vi "AODScanner_5_May_2014.vi"() -> ()   [LabVIEW 2012]
uses:
  AODAcq/AODAcq.lvclass
  <vilib>/rvi/interface/nirviReadWriteControl/nirviReadWriteControl.xnode
  FPGA_Control/AODRef.ctl
  <vilib>/rvi/interface/nirviMethod/nirviMethod.xnode
  <vilib>/rvi/errors/niLvFpgaMergeErrorWithErrorCode.vi
  Motion Stabilization/GlobalVars.vi
  <vilib>/DAQmx/write.llb/DAQmx Write (Analog DBL 1Chan 1Samp).vi
  <vilib>/DAQmx/read.llb/DAQmx Read (Analog Wfm 1Chan NSamp).vi
panel:
  out "Motion FIFO":refnum<queue>
  out "Motion ROIs":T1(array[cluster])
  out "Motion Plane Centers":i32[][](array[numeric])
  out "Number of Motion Planes":i32
  in  "Motion rate (Hz) 2":dbl=10.0
  out "error out 3":errorcluster
  out "Out Points":i32[][](array[numeric])
  out "Y-Z Motion Points":i32[][](array[numeric])
  out "X-Y Motion Points":i32[][](array[numeric])
  out "Points_um":dbl[][](array[numeric])
  out "Lens Magnification":i32=20
  in  "Matlab Server Shared Folder":string="c:\\temp"
  in  "Matlab Server IP Address":string="10.21.16.18"
  in  "External Magnification":dbl=1.3
  out "error out 2":errorcluster
  out "Objective Position":cluster{"X":dbl, "Y":dbl, "Z":dbl}
  out "Numeric":i32=299
  out "error out":errorcluster
  out "ROIs":T1(array[cluster])
  out "Histogram":dynamicdata(graph)
  out "Raw samples remaining":u32
  out "Temporal samples remaining":u32
  out "Motion samples remaining":u32
  out "Image samples remaining":u32
  out "Recording File":path
  out "Waveform Chart":waveform(dbl)(graph)
  out "Ephys":bool
  in  "TraceElements":u32=10000
  out "ScanProgress":dbl(slide) scale=0.0..1.0
  in  "Abort":bool
  out "Progress":dbl(slide) scale=0.0..1.0
  in  "SweepSettings":bool
  in  "stop":bool
  in  "Power":dbl(slide)=2.5 min=0.0 max=5.0 step=0.1 scale=0.0..2.5
  out "Scan":bool
  out "Volume":bool
  in  "Tab Control":enum32{"Setup", "Volume", "Traces", "Motion"}(tab)
  in  "Store Raw":bool
  in  "Disp Volume":bool=TRUE
  in  "Save Volume":bool
  in  "Ephys":bool
  in  "Motion rate (Hz)":dbl=10.0
  in  "Scan Settings (um)":T2={"XStart"=-100, "XEnd"=100, "XNum"=250, "YStart"=-100, "YEnd"=100, "YNum"=250, "ZStart"=-30, "ZEnd"=70, "ZNum"=60}
  in  "Objective":enum16{"20x Olympus"}(ring)
  in  "Scan Time (s)":dbl=300.0
  in  "Volume Reps":i32=1 min=1 max=10000
  in  "Volume":bool
  in  "Scan":bool
  in  "Motion Channel To Analyze":i32=2 min=1 max=2
  in  "Motion Analysis":bool
  in  "Per Cell Motion Analysis":bool
  in  "Sampling Structure":u16(ring) items=["Cube Vertices"]
  in  "Motion Box Params":T3={"XY Offset"=3, "Z Offset"=6, "Line Length"=12.0, "Box Size"=12.0}
  in  "ClearMotionCenters":bool
  in  "Point Centering":bool=TRUE
  in  "Recenter":bool caption="OK Button"
  out "Motion Points (Ch1)":u32
  out "Number selected":u32
  in  "Contrast":dbl(slide)=99.63636363636364 scale=98.0..100.0
  out "ImCh2":T4(plugin-control)
  out "ImCh1":T4(plugin-control)
  in  "Section":dbl min=0.0 max=59.0 step=1.0
  in  "Segment":bool
  out "Motion Increment":u32
  in  "Offset":dbl(slide)=0.010101010101010102 scale=0.0..1.0
  in  "ClearPoints":bool
  out "Total Motion Points":i32
  out "Motion Ch1":T4(plugin-control)
  out "Ephys":waveform(dbl)[](graph)
  out "Traces":waveform(dbl)[](graph)
  in  "Down Rate":i32=500
  in  "Spacing":dbl=100.0
  in  "Decimate":bool
  in  "Baseline Offset":dbl
  out "Motion Ch2":T4(plugin-control)
  out "Finished":bool
  out "Stopped":bool
  out "AODAcq out":refnum<class "AODAcq.lvclass">
  in  "Debug":bool
  in  "GridPoints":u16=10
  out "Scan Settings":T2
  out "VolData":i32[][](array[numeric])
  in  "VolumeElements":u32=10000
  in  "Points":i32[][](array[numeric])
  # "Off"
  # "On"
  # "On"
  # "Off"
  # "Off"
  # "On"
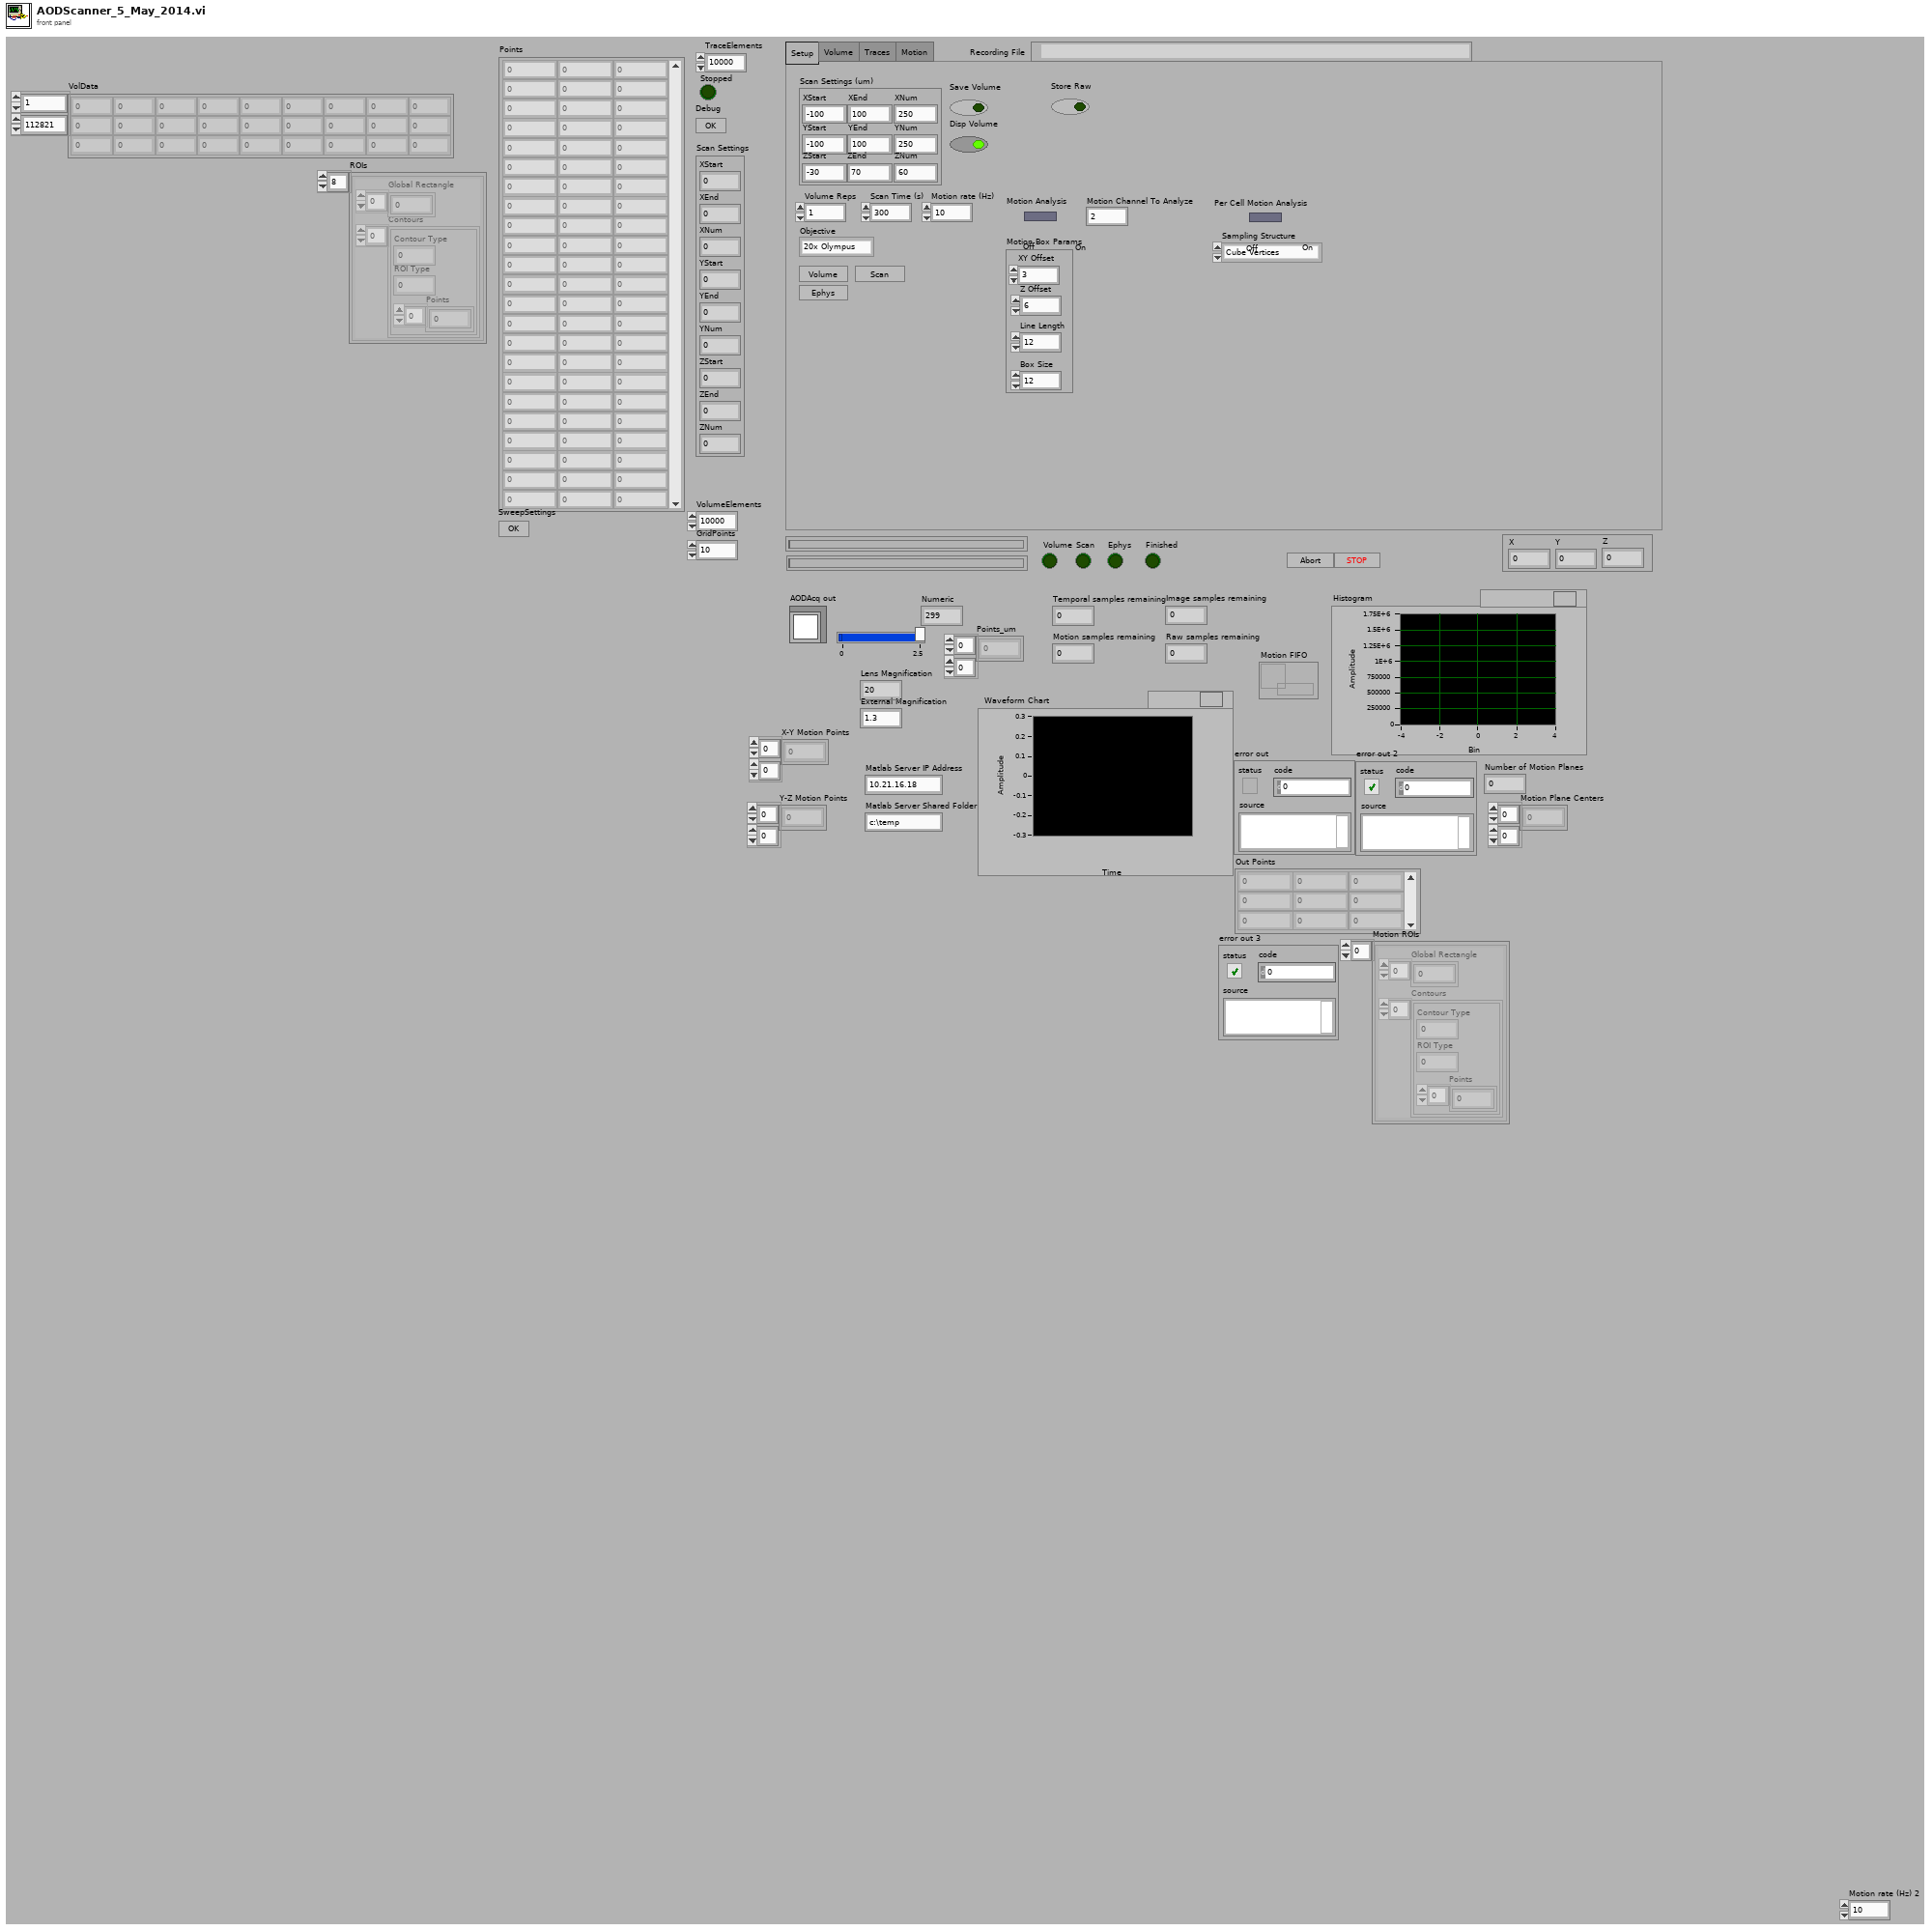
[diagram p1: front panel]
types:
  T1 = cluster{"Global Rectangle":i32[], "Contours":cluster{"Contour Type":u32, "ROI Type":u32, "Points":i32[]}[]}[]
  T2 = cluster{"XStart":i32, "XEnd":i32, "XNum":i32, "YStart":i32, "YEnd":i32, "YNum":i32, "ZStart":i32, "ZEnd":i32, "ZNum":i32}
  T3 = cluster{"XY Offset":i32, "Z Offset":i32, "Line Length":dbl, "Box Size":dbl}
  T4 = typedef "IMAQ Image.ctl" = refnum<image>
  T5 = typedef "Image Type" = u32
  T6 = cluster{"Global Rectangle":i32[], "Contours":cluster{"Contour Type":u32, "ROI Type":u32, "Points":i32[]}[]}
  T7 = cluster{"queue out":refnum<queue>, "queue out":refnum<queue>, "queue out":refnum<queue>}
  T8 = typedef "AODRef.ctl" = refnum<k20>
  T9 = cluster{"Scan Settings":cluster{"XStart":i32, "XEnd":i32, "XNum":i32, "YStart":i32, "YEnd":i32, "YNum":i32, "ZStart":i32, "ZEnd":i32, "ZNum":i32}, "Scan Settings (um)":cluster{"XStart":i32, "XEnd":i32, "XNum":i32, "YStart":i32, "YEnd":i32, "YNum":i32, "ZStart":i32, "ZEnd":i32, "ZNum":i32}}
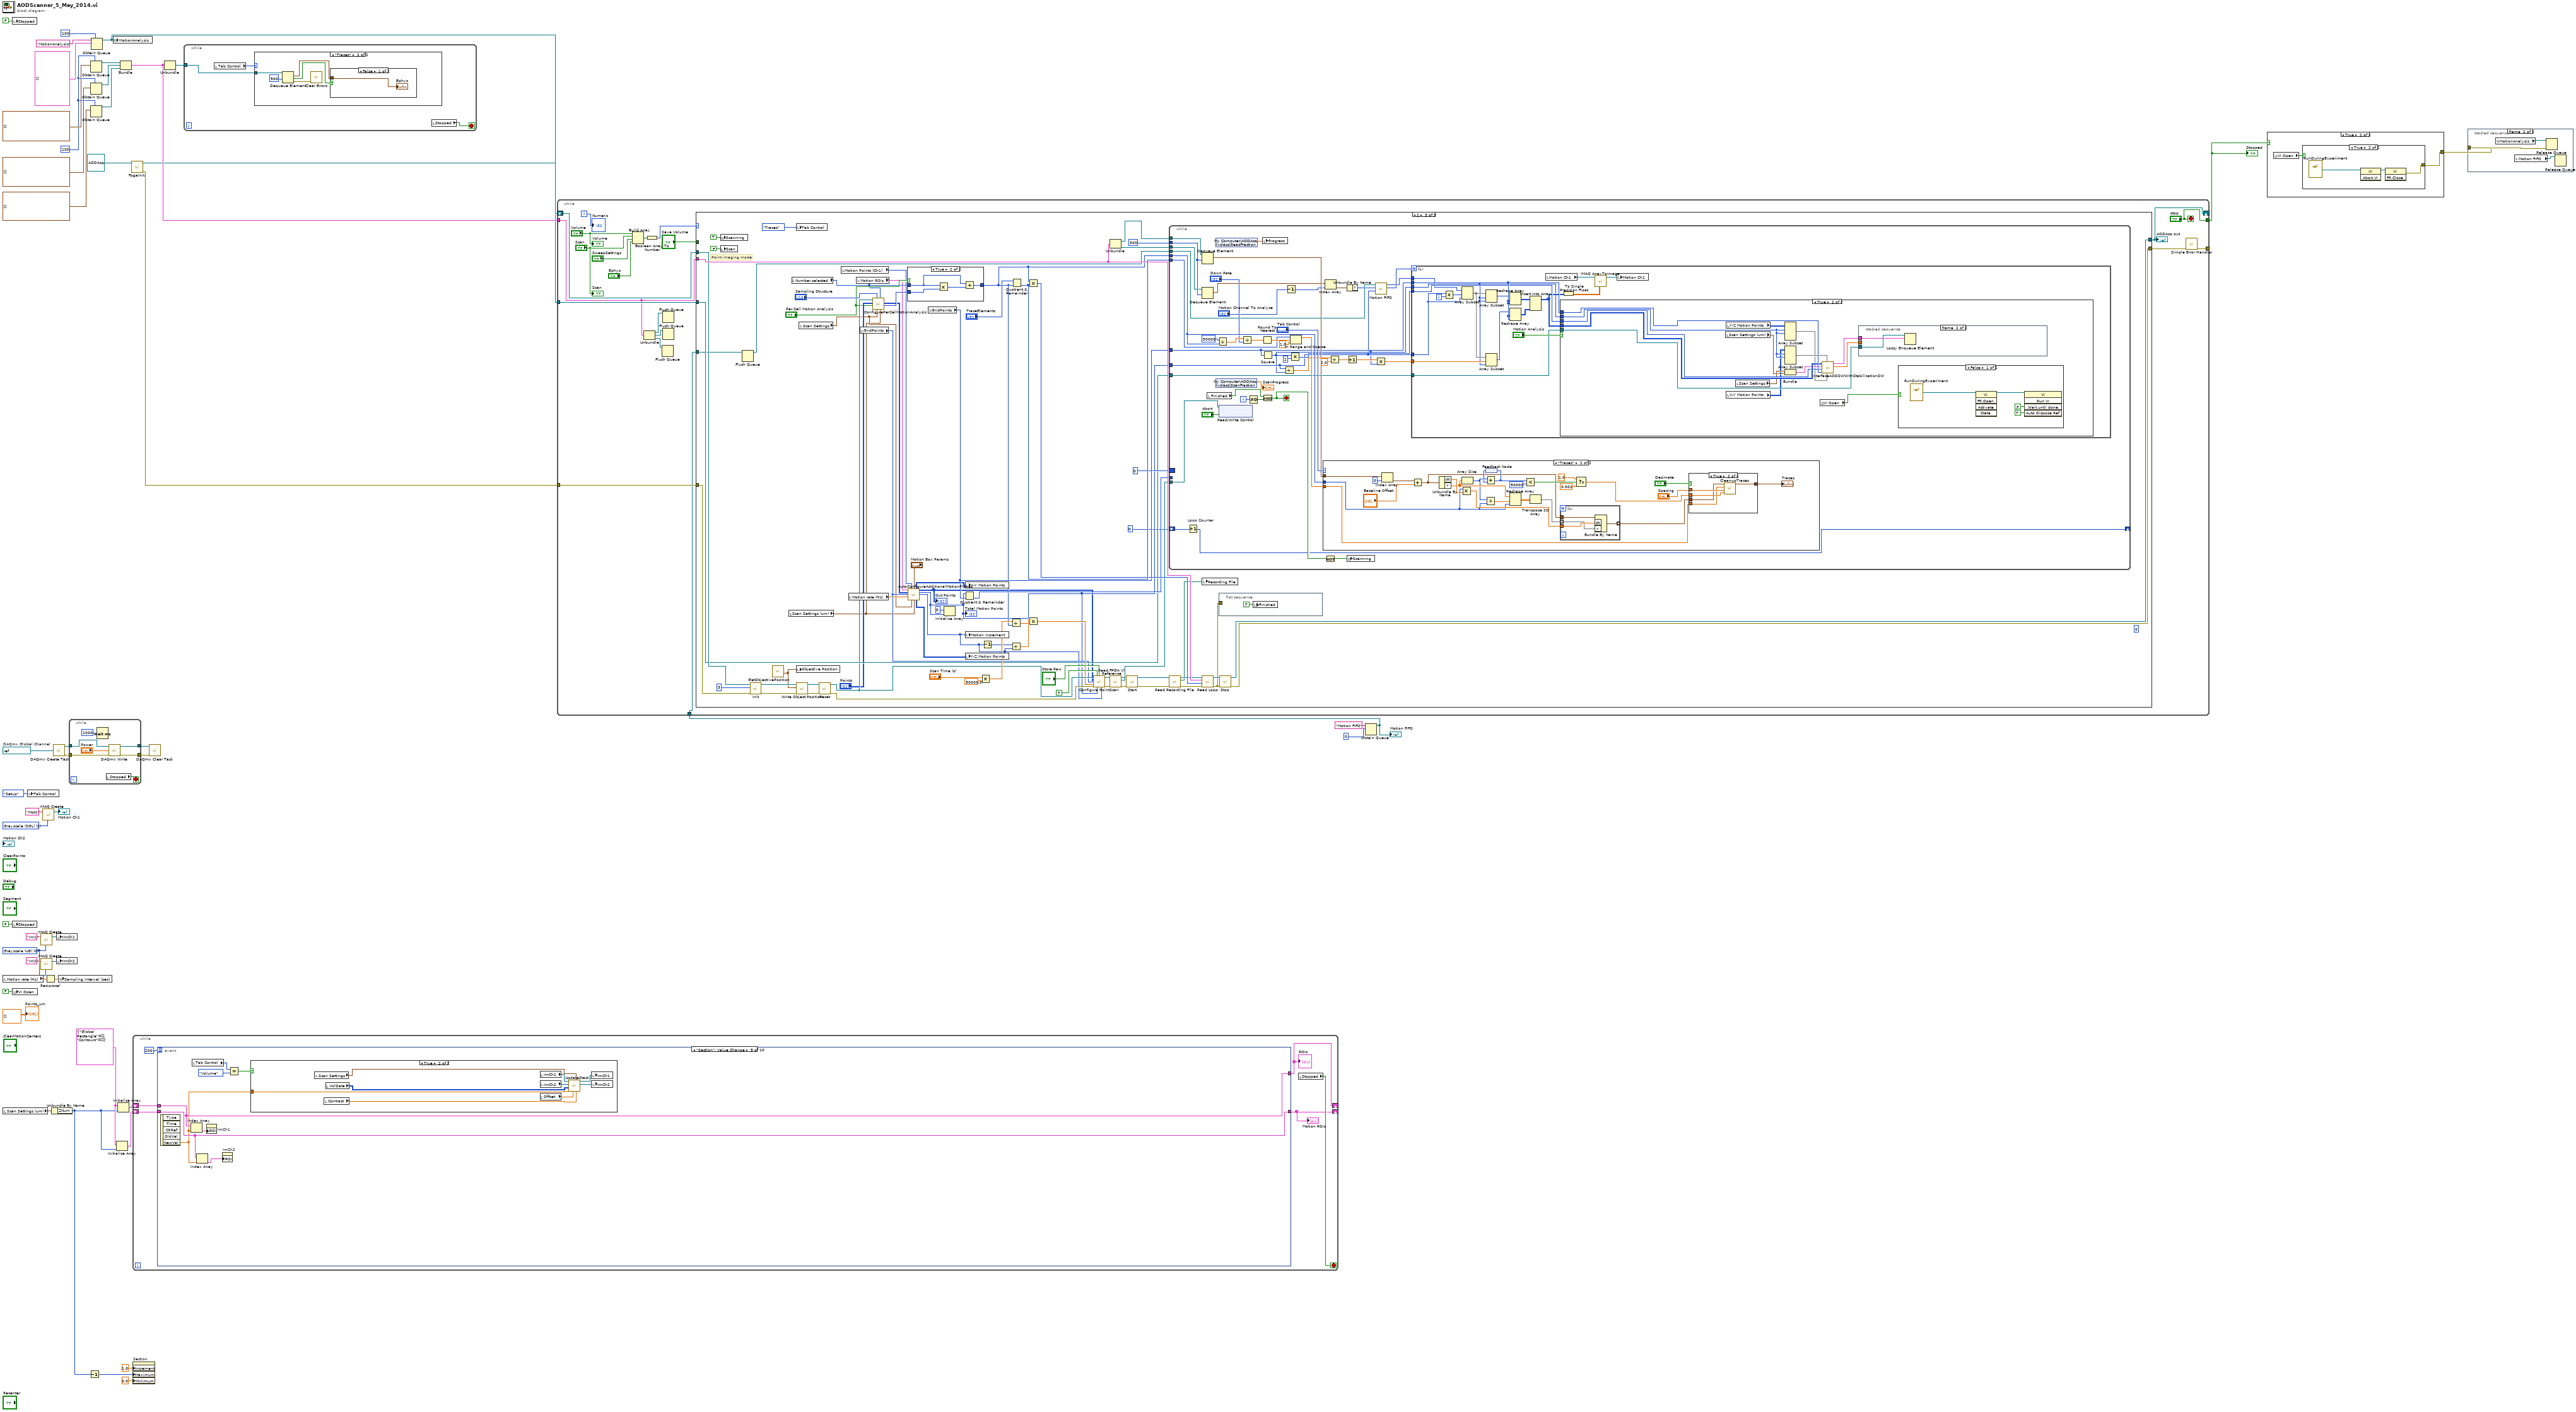
[diagram p0: block diagram]
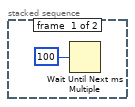
[diagram p2: hidden frame]
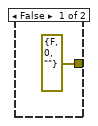
[diagram p3: hidden frame]
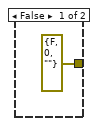
[diagram p4: hidden frame]
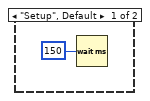
[diagram p5: hidden frame]
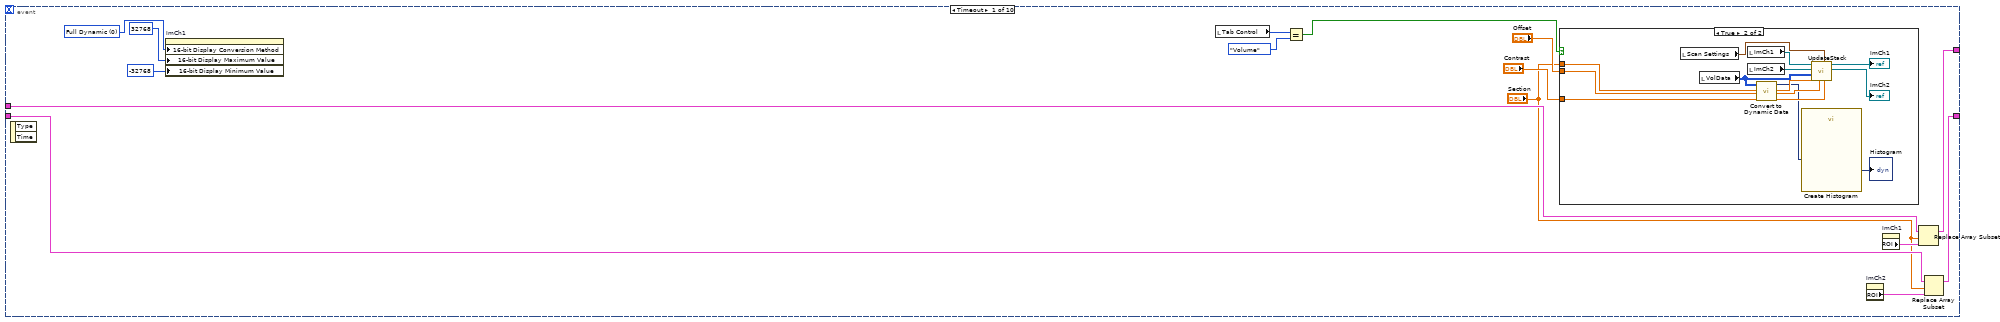
[diagram p7: hidden frame]
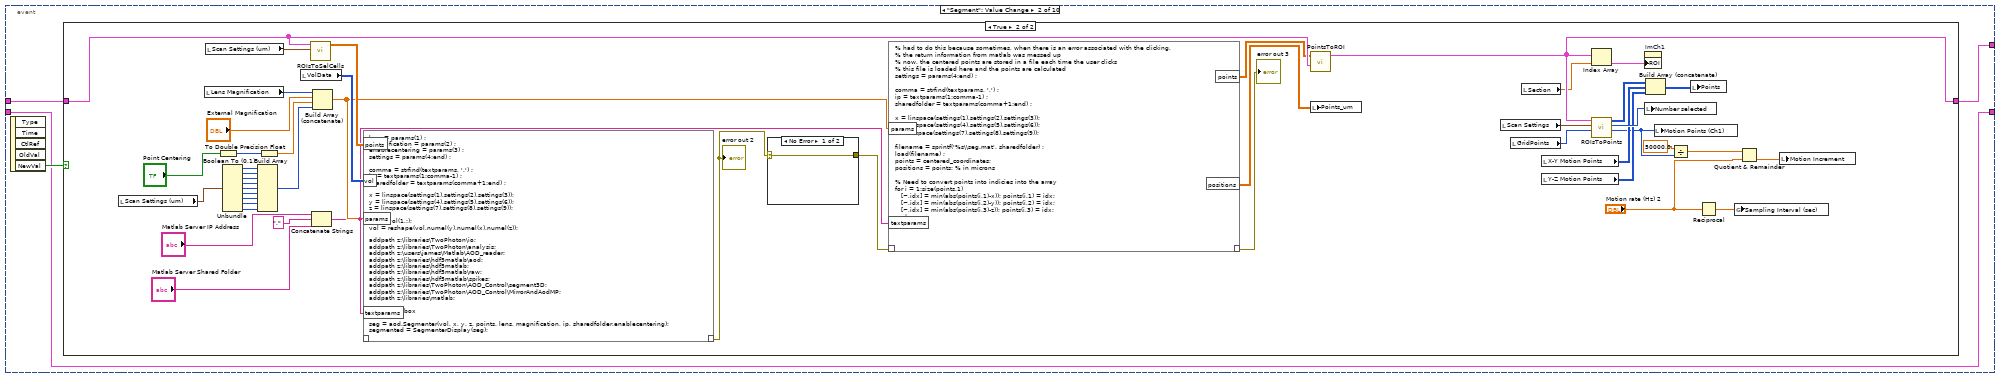
[diagram p9: hidden frame]
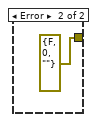
[diagram p11: hidden frame]
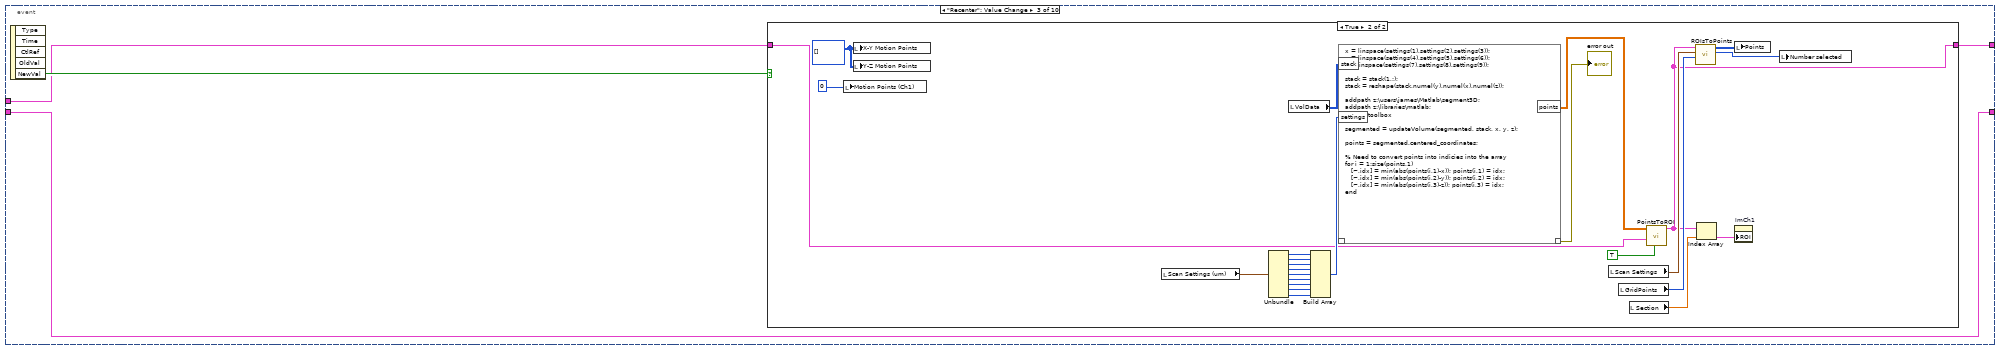
[diagram p12: hidden frame]
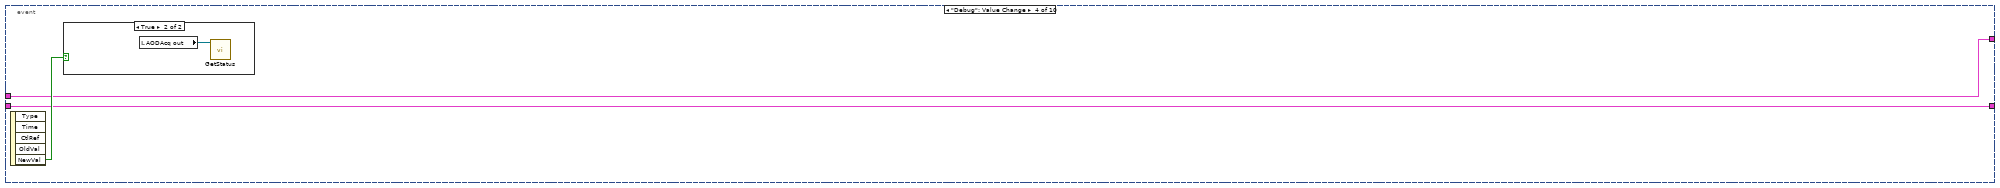
[diagram p14: hidden frame]
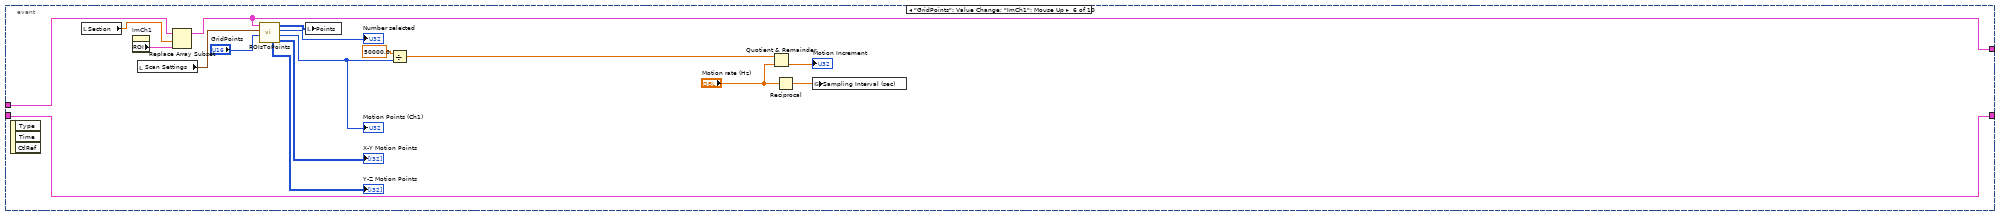
[diagram p17: hidden frame]
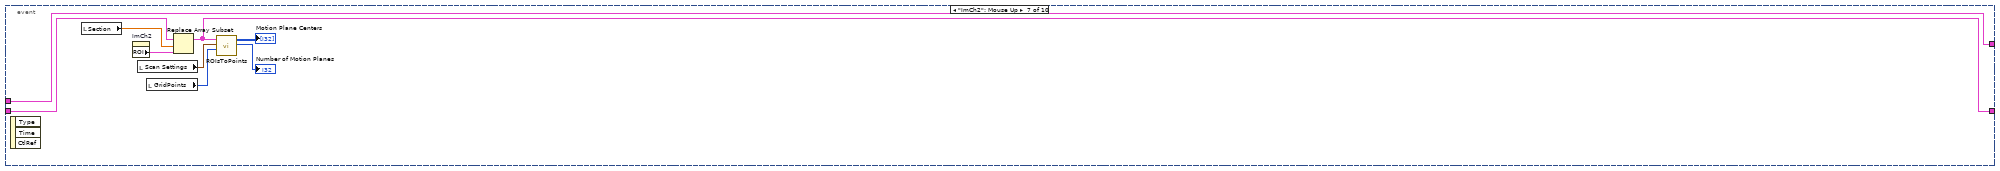
[diagram p18: hidden frame]
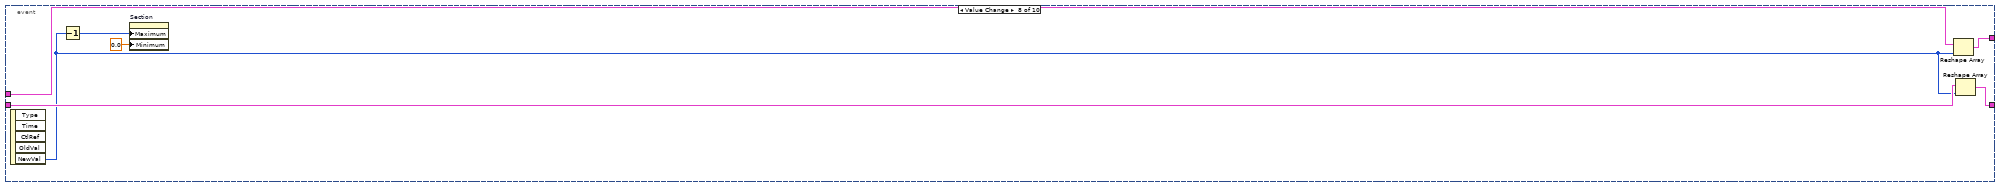
[diagram p19: hidden frame]
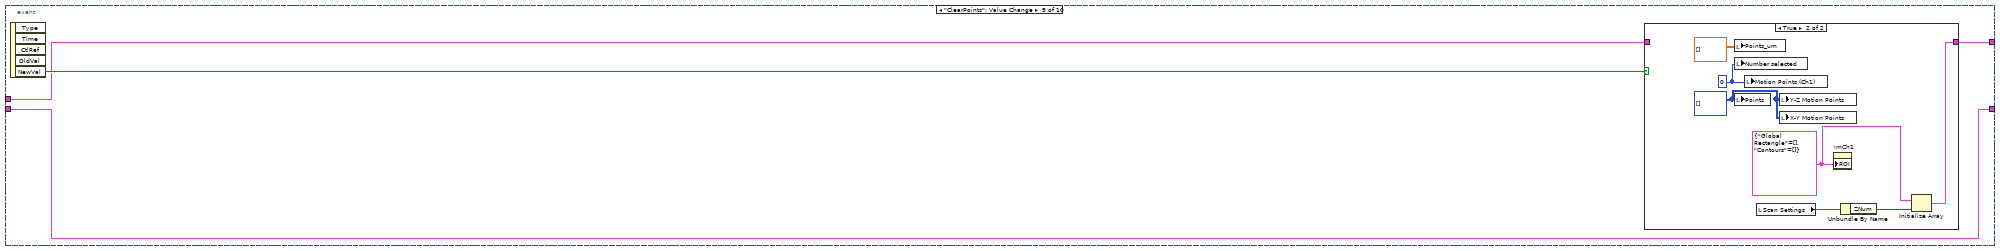
[diagram p20: hidden frame]
diagram:
  w18 = 100 ("max queue size (-1, unlimited)")
  w23 = T5 2 items=["Grayscale (U8)", "Grayscale (I16)", "Grayscale (SGL)", "Complex (CSG)", "RGB (U32)", "HSL (U32)", "RGB (U64)", "Grayscale (U16)"] ("Image Type")
  w34 = T5 0 items=["Grayscale (U8)", "Grayscale (I16)", "Grayscale (SGL)", "Complex (CSG)", "RGB (U32)", "HSL (U32)", "RGB (U64)", "Grayscale (U16)"] ("Image Type")
  w6 = T6 {"Global Rectangle"=[], "Contours"=[]} ("ROI")
  w44 = refnum<k21> "AOD Gain"  # DAQmx Global Channel
  n1 = local read "Motion rate (Hz)"() -> (w9:dbl)
  n2 = local read "Scan Settings (um)"() -> (w38:T2)
  n3 = local write "Stopped"(FALSE ("Stopped")) -> ()
  n4 = local write "Stopped"(FALSE ("Stopped")) -> ()
  n5 = global write "GlobalVars.vi" "VI Open"(FALSE ("VI Open")) -> ()
  n6 = local write "Tab Control"(enum32{"Setup", "Volume", "Traces", "Motion"}."Setup" ("Tab Control")) -> ()
  n7 = call "IMAQ Create"("Image Name"="Im1", "Image Type"=w34) -> ("New Image"=w46:T4)  [unwired: 3 in, 1 out]
  n8 = call "IMAQ Create"("Image Name"="Im2", "Image Type"=w34) -> ("New Image"=w45:T4)  [unwired: 3 in, 1 out]
  n9 = call "IMAQ Create"("Image Name"="Mot1", "Image Type"=w23) -> ("New Image"=→"Motion Ch1":T4)  [unwired: 3 in, 1 out]
  n10 = Reciprocal(x=w9) -> (1/x=w8:dbl)
  n11 = Unbundle By Name(w38) -> ("ZNum"=w5:i32)
  n12 = call <vilib>:"DAQmx Create Task.vi"("global virtual channels"=w44) -> ("task out"=w43:refnum<k21>, "error out"=w42:errorcluster)  [unwired: 4 in, 9 out]
  n13 = local write "ImCh1"(w46) -> ()
  n14 = local write "ImCh2"(w45) -> ()
  n15 = global write "GlobalVars.vi" "Sampling Interval (sec)"(w8) -> ()
  n16 = while {
    tunnel: w43 -> [w55]
    tunnel: w42 -> [w54]
    tunnel: [w53] -> w41
    tunnel: [w52] -> w40
    stop <- w51 stop-if-true
    n17 = Wait (ms)(milliseconds to wait=u32 1000) -> ()  [unwired: 1 out]
    n18 = local read "Stopped"() -> (w51:bool)
    n19 = call-poly <vilib>:"DAQmx Write.vi"("task/channels in"=w55, "data"="Power", "error in"=w54) -> ("task out"=w53:refnum<k21>, "error out"=w52:errorcluster)  [unwired: 10 in, 1 out]
  }
  n20 = Decrement(x=w5) -> (x-1=w33:i32)
  n21 = Obtain Queue(max queue size (-1, unlimited)=w18, element data type=waveform(i32)[] []) -> (queue out=w29:refnum<queue>)  [unwired: 3 in, 2 out]
  n22 = Obtain Queue(max queue size (-1, unlimited)=w18, element data type=waveform(dbl)[] []) -> (queue out=w30:refnum<queue>)  [unwired: 3 in, 2 out]
  n23 = Obtain Queue(max queue size (-1, unlimited)=w18, element data type=waveform(i32)[] []) -> (queue out=w28:refnum<queue>)  [unwired: 3 in, 2 out]
  n24 = Obtain Queue(max queue size (-1, unlimited)=100, name (unnamed)="MotionAnalysis", element data type=cluster{dbl[][], dbl, dbl, dbl, dbl, dbl, dbl}[] [] ("Array 2")) -> (queue out=w12:refnum<queue>)  [unwired: 2 in, 2 out]
  n25 = global write "GlobalVars.vi" "MotionAnalysis"(w12) -> ()
  n26 = Initialize Array(w6, w5) -> (w4:T1)
  n27 = Initialize Array(w6, w5) -> (w37:T1)
  n28 = Bundle("queue out"=w29, "queue out"=w30, "queue out"=w28) -> (w27:T7)  [unwired: 1 in]
  n29 = call-dynamic "FpgaInit.vi"("AODAcq in"=refnum<class "AODAcq.lvclass"> refnum ("AODAcq.lvclass")) -> ("error out"=w21:errorcluster, "AODAcq out"=w20:refnum<class "AODAcq.lvclass">)  [unwired: 9 in]
  n30 = while {
    shift-right: [w61] -> _
    shift-left: w37 -> [w62]
    shift-right: [w58] -> _
    shift-left: w4 -> [w57]
    stop <- w59 stop-if-true
    n31 = event shown="[4] \"Section\": Value Change" {
      selector: _ -> [_ _ _ _ _ _ _ _ _ _]
      dyn-events: _ -> [_ _ _ _ _ _ _ _ _ _]
      timeout: 200 -> [_ _ _ _ _ _ _ _ _ _]
      tunnel: w62 -> [w76 w91 w143 w173 w182 w209 w210 w223 w227 w239]
      tunnel: [w77 w90 w144 w173 w182 w206 w210 w222 w228 w239] -> w61
      tunnel: [w63 w89 w142 w172 w177 w193 w211 w219 w226 w240] -> w58
      tunnel: w57 -> [w66 w89 w142 w172 w177 w193 w216 w221 w226 w238]
      event Timeout {
        w71 = u32 0 items=["Full Dynamic", "Downshift", "Given Range", "90% Dynamic", "Given Percent Range"] ("16-bit Display Mapping:Conversion Method")
        n32 = event-data() -> ()  [unwired: 1 in, 2 out]
        n33 = property on="ImCh1" class="ImageControl"("16-bit Display Conversion Method"=w71, "16-bit Display Maximum Value"=32768 ("16-bit Display Mapping:Maximum Value"), "16-bit Display Minimum Value"=-32768 ("16-bit Display Mapping:Maximum Value")) -> ()  [unwired: 2 in, 2 out]
        n34 = local read "Tab Control"() -> (w74:enum32{"Setup", "Volume", "Traces", "Motion"})
        n35 = Equal?(x=w74, y=enum32{"Setup", "Volume", "Traces"}."Volume") -> (x = y?=w72:bool)
        n36 = case shown="True" w72 {
          tunnel: "Section" -> [_ w83]
          tunnel: "Offset" -> [_ w82]
          tunnel: "Contrast" -> [_ w81]
          frame False {
          }
          frame True {
            n37 = local read "Scan Settings"() -> (w84:T2)
            n38 = local read "VolData"() -> (w80:i32[][])
            n39 = local read "ImCh1"() -> (w88:T4)
            n40 = local read "ImCh2"() -> (w87:T4)
            n41 = call "Convert to Dynamic Data"("2D Array"=w80) -> ("Dynamic Data Type"=w79:dynamicdata)  [unwired: 3 in]
            n42 = call "Create Histogram"("Signal"=w79) -> ("Histogram"=→"Histogram":dynamicdata)  [unwired: 9 in, 1 out]
            n43 = call "UpdateStack.vi"("Contrast"=w81, "Scan Settings"=w84, "Offset"=w82, "Section"=w83, "ImData"=w80, "Im2 2"=w87, "Im1 In"=w88) -> ("Im2 Out"=→"ImCh2":T4, "Im1 Out"=→"ImCh1":T4)  [unwired: 3 in]
          }
        }
        n44 = property on="ImCh2" class="ImageControl"() -> ("ROI"=w65:T6)  [unwired: 2 in, 2 out]
        n45 = property on="ImCh1" class="ImageControl"() -> ("ROI"=w75:T6)  [unwired: 2 in, 2 out]
        n46 = Replace Array Subset(array=w76, new element=w75, index="Section") -> (w77:T1)
        n47 = Replace Array Subset(array=w66, new element=w65, index="Section") -> (w63:T1)
      }
      event "Segment": Value Change {
        n48 = event-data() -> ("NewVal"=w92:bool)  [unwired: 1 in, 4 out]
        n49 = case shown="True" w92 {
          tunnel: w91 -> [w93 w117]
          tunnel: [w93 w125] -> w90
          frame False {
          }
          frame True {
            n50 = local read "Scan Settings (um)"() -> (w139:T2)
            n51 = local read "Lens Magnification"() -> (w113:i32)
            n52 = local read "Scan Settings (um)"() -> (w115:T2)
            n53 = Boolean To (0,1)(Boolean="Point Centering") -> (0, 1=w118:i16)
            n54 = Unbundle(w139) -> ("XStart"=w138:i32, "XEnd"=w137:i32, "XNum"=w136:i32, "YStart"=w135:i32, "YEnd"=w134:i32, "YNum"=w133:i32, "ZStart"=w132:i32, "ZEnd"=w131:i32, "ZNum"=w130:i32)
            n55 = Build Array(w138, w137, w136, w135, w134, w133, w132, w131, w130) -> (w107:i32[])
            n56 = To Double Precision Float(number=w118) -> (double precision float=w111:dbl)
            n57 = local read "VolData"() -> (w129:i32[][])
            n58 = call "ROIsToSelCells.vi"("Scan Settings"=w115, "ROI"=w117) -> ("Points_um"=w114:dbl[][])  [unwired: 8 in, 1 out]
            n59 = Concatenate Strings("Matlab Server IP Address", "," ("string"), "Matlab Server Shared Folder") -> (w103:string)
            n60 = Build Array (concatenate)(w113, "External Magnification", w111, w107) -> (w104:dbl[])
            n61 = script code="lens = params(1) ;\nmagnification = params(2) ;\nenablecentering = params(3) ;\nsettings = params(4:end) ;\n\ncomma = strfind(textparams, ',') ;\nip = textparams(1:comma-1) ;\nsharedfolder = textparams(comma+1:end) ;\n\nx = linspace(settings(1),settings(2),settings(3));\ny = linspace(settings(4),settings(5),settings(6));\nz = linspace(settings(7),settings(8),settings(9));\n\nvol = vol(1,:);\nvol = reshape(vol,numel(y),numel(x),numel(z));\n\naddpath z:\\libraries\\TwoPhoton\\io;\naddpath z:\\libraries\\TwoPhoton\\analysis;\naddpath z:\\users\\james\\Matlab\\AOD_reader;\naddpath z:\\libraries\\hdf5matlab\\aod;\naddpath z:\\libraries\\hdf5matlab;\naddpath z:\\libraries\\hdf5matlab\\raw;\naddpath z:\\libraries\\hdf5matlab\\spikes;\naddpath z:\\libraries\\TwoPhoton\\AOD_Control\\segment3D;\naddpath z:\\libraries\\TwoPhoton\\AOD_Control\\MirrorAndAodMP;\naddpath z:\\libraries\\matlab;\n\nrehash toolbox\n\nseg = aod.Segmenter(vol, x, y, z, points, lens, magnification, ip, sharedfolder,enablecentering);\nsegmented = SegmenterDisplay(seg);"("vol"=w129, "params"=w104, "textparams"=w103, "points"=w114) -> ("??"=w101:errorcluster)  [unwired: 1 in]
            "error out 2" <- w101
            n62 = case shown="No Error" w101 {
              selector: w101 -> [w140 _]
              tunnel: [w140 errorcluster {"status"=FALSE, "code"=0, "source"=""} ("error IO")] -> w100
              frame No Error {
              }
              frame Error {
              }
            }
            n63 = script code="% had to do this because sometimes, when there is an error associated with the clicking,\n% the return information from matlab was messed up\n% now, the centered points are stored in a file each time the user clicks\n% this file is loaded here and the points are calculated\nsettings = params(4:end) ;\n\ncomma = strfind(textparams, ',') ;\nip = textparams(1:comma-1) ;\nsharedfolder = textparams(comma+1:end) ;\n\nx = linspace(settings(1),settings(2),settings(3));\ny = linspace(settings(4),settings(5),settings(6));\nz = linspace(settings(7),settings(8),settings(9));\n\nfilename = sprintf('%s\\\\seg.mat', sharedfolder) ;\nload(filename) ;\npoints = centered_coordinates;\npositions = points; % in microns\n\n% Need to convert points into indicies into the array\nfor i = 1:size(points,1)\n   [~,idx] = min(abs(points(i,1)-x)); points(i,1) = idx;\n   [~,idx] = min(abs(points(i,2)-y)); points(i,2) = idx;\n   [~,idx] = min(abs(points(i,3)-z)); points(i,3) = idx;\nend"("??"=w100, "params"=w104, "textparams"=w103) -> ("??"=→"error out 3":errorcluster, "points"=w106:dbl[][], "positions"=w105:dbl[][])
            n64 = call "PointsToROI.vi"("Old ROIs"=w117, "Points"=w106) -> ("ROIs"=w125:T1)  [unwired: 9 in]
            n65 = local write "Points_um"(w105) -> ()
            n66 = local read "Scan Settings"() -> (w127:T2)
            n67 = local read "GridPoints"() -> (w116:u16)
            n68 = local read "Section"() -> (w124:dbl)
            n69 = local read "X-Y Motion Points"() -> (w121:i32[][])
            n70 = local read "Y-Z Motion Points"() -> (w120:i32[][])
            n71 = Index Array(array=w125, index=w124) -> (element=w126:T6)
            n72 = call "ROIsToPoints.vi"("GridPoints"=w116, "Scan Settings"=w127, "ROI"=w125) -> ("Number of motion points"=w94:i32, "Number of points"=w128:i32, "Points"=w123:i32[][])  [unwired: 4 in, 2 out]
            n73 = property on="ImCh1" class="ImageControl"("ROI"=w126) -> ()  [unwired: 2 in, 2 out]
            n74 = local write "Number selected"(w128) -> ()
            n75 = Build Array (concatenate)(w123, w121, w120) -> (w122:i32[][])
            n76 = local write "Motion Points (Ch1)"(w94) -> ()
            n77 = Divide(x=50000.0, y=w94) -> (x/y=w96:dbl)
            n78 = local write "Points"(w122) -> ()
            n79 = Reciprocal(x="Motion rate (Hz) 2") -> (1/x=w97:dbl)
            n80 = global write "GlobalVars.vi" "Sampling Interval (sec)"(w97) -> ()
            n81 = Quotient & Remainder(x=w96, y="Motion rate (Hz) 2") -> (floor(x/y)=w95:dbl)  [unwired: 1 out]
            n82 = local write "Motion Increment"(w95) -> ()
          }
        }
      }
      event "Recenter": Value Change {
        n83 = event-data() -> ("NewVal"=w145:bool)  [unwired: 1 in, 4 out]
        n84 = case shown="True" w145 {
          tunnel: [w146 w151] -> w144
          tunnel: w143 -> [w146 w154]
          frame False {
          }
          frame True {
            w149 = i32[][] [] ("Points")
            n85 = local write "Motion Points (Ch1)"(u32 0 ("Number of Motion Points")) -> ()
            n86 = local write "X-Y Motion Points"(w149) -> ()
            n87 = local write "Y-Z Motion Points"(w149) -> ()
            n88 = local read "Scan Settings (um)"() -> (w157:T2)
            n89 = Unbundle(w157) -> ("XStart"=w171:i32, "XEnd"=w170:i32, "XNum"=w169:i32, "YStart"=w168:i32, "YEnd"=w167:i32, "YNum"=w166:i32, "ZStart"=w165:i32, "ZEnd"=w164:i32, "ZNum"=w163:i32)
            n90 = local read "VolData"() -> (w161:i32[][])
            n91 = Build Array(w171, w170, w169, w168, w167, w166, w165, w164, w163) -> (w162:i32[])
            n92 = script code="x = linspace(settings(1),settings(2),settings(3));\ny = linspace(settings(4),settings(5),settings(6));\nz = linspace(settings(7),settings(8),settings(9));\n\nstack = stack(1,:);\nstack = reshape(stack,numel(y),numel(x),numel(z));\n\naddpath z:\\users\\james\\Matlab\\segment3D;\naddpath z:\\libraries\\matlab;\nrehash toolbox\n\nsegmented = updateVolume(segmented, stack, x, y, z);\n\npoints = segmented.centered_coordinates;\n\n% Need to convert points into indicies into the array\nfor i = 1:size(points,1)\n   [~,idx] = min(abs(points(i,1)-x)); points(i,1) = idx;\n   [~,idx] = min(abs(points(i,2)-y)); points(i,2) = idx;\n   [~,idx] = min(abs(points(i,3)-z)); points(i,3) = idx;\nend"("stack"=w161, "settings"=w162) -> ("??"=→"error out":errorcluster, "points"=w160:dbl[][])  [unwired: 1 in]
            n93 = local read "Scan Settings"() -> (w156:T2)
            n94 = local read "GridPoints"() -> (w158:u16)
            n95 = local read "Section"() -> (w152:dbl)
            n96 = call "PointsToROI.vi"("Clear Motion Planes"=TRUE, "Old ROIs"=w154, "Points"=w160) -> ("ROIs"=w151:T1)  [unwired: 8 in]
            n97 = call "ROIsToPoints.vi"("GridPoints"=w158, "Scan Settings"=w156, "ROI"=w151) -> ("Number of points"=w159:i32, "Points"=w150:i32[][])  [unwired: 4 in, 3 out]
            n98 = Index Array(array=w151, index=w152) -> (element=w153:T6)
            n99 = local write "Points"(w150) -> ()
            n100 = property on="ImCh1" class="ImageControl"("ROI"=w153) -> ()  [unwired: 2 in, 2 out]
            n101 = local write "Number selected"(w159) -> ()
          }
        }
      }
      event "Debug": Value Change {
        n102 = event-data() -> ("NewVal"=w174:bool)  [unwired: 1 in, 4 out]
        n103 = case shown="True" w174 {
          frame False {
          }
          frame True {
            n104 = local read "AODAcq out"() -> (w175:refnum<class "AODAcq.lvclass">)
            n105 = call-dynamic "GetStatus.vi"("AODAcq in"=w175) -> ()  [unwired: 8 in, 3 out]
          }
        }
      }
      event "Section": Value Change {
        n106 = event-data() -> ("NewVal"=w176:dbl)  [unwired: 1 in, 4 out]
        n107 = Index Array(array=w182, index=w176) -> (element=w183:T6)
        n108 = local read "Tab Control"() -> (w181:enum32{"Setup", "Volume", "Traces", "Motion"})
        n109 = Index Array(array=w177, index=w176) -> (element=w178:T6)
        n110 = property on="ImCh1" class="ImageControl"("ROI"=w183) -> ()  [unwired: 2 in, 2 out]
        n111 = property on="ImCh2" class="ImageControl"("ROI"=w178) -> ()  [unwired: 2 in, 2 out]
        n112 = Equal?(x=w181, y=enum32{"Setup", "Volume", "Traces"}."Volume") -> (x = y?=w179:bool)
        n113 = case shown="True" w179 {
          tunnel: w176 -> [_ w187]
          frame False {
          }
          frame True {
            n114 = local read "Scan Settings"() -> (w186:T2)
            n115 = local read "Contrast"() -> (w184:dbl)
            n116 = local read "VolData"() -> (w192:i32[][])
            n117 = local read "ImCh1"() -> (w190:T4)
            n118 = local read "ImCh2"() -> (w191:T4)
            n119 = local read "Offset"() -> (w185:dbl)
            n120 = call "UpdateStack.vi"("Contrast"=w184, "Scan Settings"=w186, "Offset"=w185, "Section"=w187, "ImData"=w192, "Im2 2"=w191, "Im1 In"=w190) -> ("Im2 Out"=w189:T4, "Im1 Out"=w188:T4)  [unwired: 3 in]
            n121 = local write "ImCh1"(w188) -> ()
            n122 = local write "ImCh2"(w189) -> ()
          }
        }
      }
      event "GridPoints": Value Change; "ImCh1": Mouse Up {
        n123 = event-data() -> ()  [unwired: 1 in, 3 out]
        n124 = local read "Section"() -> (w207:dbl)
        n125 = property on="ImCh1" class="ImageControl"() -> ("ROI"=w208:T6)  [unwired: 2 in, 2 out]
        n126 = local read "Scan Settings"() -> (w205:T2)
        n127 = Replace Array Subset(array=w209, new element=w208, index=w207) -> (w206:T1)
        n128 = call "ROIsToPoints.vi"("GridPoints"="GridPoints", "Scan Settings"=w205, "ROI"=w206) -> ("X-Y Motion Points"=→"X-Y Motion Points":i32[][], "Number of motion points"=w200:i32, "Number of points"=→"Number selected":i32, "Points"=w203:i32[][], "Y-Z Motion Points"=→"Y-Z Motion Points":i32[][])  [unwired: 4 in]
        "Motion Points (Ch1)" <- w200
        n129 = local write "Points"(w203) -> ()
        n130 = Divide(x=50000.0, y=w200) -> (x/y=w199:dbl)
        n131 = Quotient & Remainder(x=w199, y="Motion rate (Hz)") -> (floor(x/y)=→"Motion Increment":dbl)  [unwired: 1 out]
        n132 = Reciprocal(x="Motion rate (Hz)") -> (1/x=w196:dbl)
        n133 = global write "GlobalVars.vi" "Sampling Interval (sec)"(w196) -> ()
      }
      event "ImCh2": Mouse Up {
        n134 = event-data() -> ()  [unwired: 1 in, 3 out]
        n135 = local read "Section"() -> (w217:dbl)
        n136 = property on="ImCh2" class="ImageControl"() -> ("ROI"=w218:T6)  [unwired: 2 in, 2 out]
        n137 = local read "Scan Settings"() -> (w215:T2)
        n138 = local read "GridPoints"() -> (w214:u16)
        n139 = Replace Array Subset(array=w216, new element=w218, index=w217) -> (w211:T1)
        n140 = call "ROIsToPoints.vi"("GridPoints"=w214, "Scan Settings"=w215, "ROI"=w211) -> ("Number of points"=→"Number of Motion Planes":i32, "Points"=→"Motion Plane Centers":i32[][])  [unwired: 4 in, 3 out]
      }
      event "Scan Settings (um).ZNum": Value Change {
        n141 = event-data() -> ("NewVal"=w220:i32)  [unwired: 1 in, 4 out]
        n142 = Decrement(x=w220) -> (x-1=w224:i32)
        n143 = property on="Section" class="DigNum (strict)"("Maximum"=w224, "Minimum"=0.0 ("Data Entry Limits:Minimum")) -> ()  [unwired: 2 in, 2 out]
        n144 = Reshape Array(w223, w220) -> (w222:T1)
        n145 = Reshape Array(w221, w220) -> (w219:T1)
      }
      event "ClearPoints": Value Change {
        n146 = event-data() -> ("NewVal"=w229:bool)  [unwired: 1 in, 4 out]
        n147 = case shown="True" w229 {
          tunnel: [w230 w237] -> w228
          tunnel: w227 -> [w230 _]
          frame False {
          }
          frame True {
            w231 = u32 0 ("Number of Motion Points")
            w232 = i32[][] [] ("Points")
            w236 = T6 {"Global Rectangle"=[], "Contours"=[]} ("ROI")
            n148 = local write "Points_um"(dbl[][] [] ("Points_um")) -> ()
            n149 = local write "Number selected"(w231) -> ()
            n150 = local write "Points"(w232) -> ()
            n151 = local write "Motion Points (Ch1)"(w231) -> ()
            n152 = local read "Scan Settings"() -> (w235:T2)
            n153 = local write "Y-Z Motion Points"(w232) -> ()
            n154 = local write "X-Y Motion Points"(w232) -> ()
            n155 = property on="ImCh1" class="ImageControl"("ROI"=w236) -> ()  [unwired: 2 in, 2 out]
            n156 = Unbundle By Name(w235) -> ("ZNum"=w234:i32)
            n157 = Initialize Array(w236, w234) -> (w237:T1)
          }
        }
      }
      event "ClearMotionCenters": Value Change {
        n158 = event-data() -> ("NewVal"=w241:bool)  [unwired: 1 in, 4 out]
        n159 = case shown="True" w241 {
          tunnel: [w242 w243] -> w240
          tunnel: w238 -> [w242 _]
          frame False {
          }
          frame True {
            w244 = T6 {"Global Rectangle"=[], "Contours"=[]} ("ROI")
            n160 = local read "Scan Settings"() -> (w246:T2)
            n161 = Unbundle By Name(w246) -> ("ZNum"=w245:i32)
            n162 = property on="ImCh2" class="ImageControl"("ROI"=w244) -> ()  [unwired: 2 in, 2 out]
            n163 = Initialize Array(w244, w245) -> (w243:T1)
          }
        }
      }
    }
    "ROIs" <- w61
    "Motion ROIs" <- w58
    n164 = local read "Stopped"() -> (w59:bool)
  }
  n165 = property on="Section" class="DigNum (strict)"("Increment"=1.0 ("Data Entry Limits:Increment"), "Maximum"=w33, "Minimum"=0.0 ("Data Entry Limits:Minimum")) -> ()  [unwired: 2 in, 2 out]
  n166 = call <vilib>:"DAQmx Clear Task.vi"("task in"=w41, "error in"=w40) -> ()  [unwired: 13 in, 1 out]
  n167 = Unbundle(w27) -> ("queue out"=w26:refnum<queue>)  [unwired: 2 out]
  n168 = while {
    tunnel: w26 -> [w249]
    stop <- w248 stop-if-true
    n169 = local read "Tab Control"() -> (w247:enum32{"Setup", "Volume", "Traces", "Motion"})
    n170 = case shown="\"Traces\"" w247 {
      tunnel: w249 -> [_ w255]
      frame "Setup", Default {
        n171 = Wait (ms)(milliseconds to wait=u32 150) -> ()  [unwired: 1 out]
      }
      frame "Traces" {
        n172 = Dequeue Element(queue=w255, timeout in ms (-1)=500) -> (element=w252:waveform(dbl)[], timed out?=w251:bool, error out=w253:errorcluster)  [unwired: 1 in, 1 out]
        n173 = call <vilib>:"Clear Errors.vi"("error in (no error)"=w253) -> ()  [unwired: 6 in, 1 out]
        n174 = case shown="False" w251 {
          tunnel: w252 -> [w256 _]
          frame False {
            "Ephys" <- w256
          }
          frame True {
          }
        }
      }
    }
    n175 = local read "Stopped"() -> (w248:bool)
  }
  n176 = Obtain Queue(name (unnamed)="Motion FIFO", element data type=0) -> (queue out=w1:refnum<queue>)  [unwired: 3 in, 2 out]
  "Motion FIFO" <- w1
  n177 = while {
    shift-right: [w270] -> _
    shift-left: w20 -> [w276]
    tunnel: w27 -> [w260]
    tunnel: w21 -> [w275]
    tunnel: [w268] -> _
    tunnel: ["stop"] -> w10
    tunnel: w12 -> [w262]
    tunnel: w1 -> [w261]
    i -> [w263]
    stop <- "stop" stop-if-true
    n178 = Build Array("Volume", "Scan", "SweepSettings", "Ephys") -> (w272:bool[])
    n179 = Unbundle(w260) -> ("queue out"=w259:refnum<queue>, "queue out"=w258:refnum<queue>, "queue out"=w257:refnum<queue>)
    n180 = Boolean Array To Number(Boolean array=w272) -> (number=w271:u32)
    n181 = Flush Queue(queue=w257) -> ()  [unwired: 1 in, 3 out]
    n182 = Flush Queue(queue=w258) -> ()  [unwired: 1 in, 3 out]
    n183 = Flush Queue(queue=w259) -> ()  [unwired: 1 in, 3 out]
    n184 = case shown="2" w271 {
      tunnel: w276 -> [w286 w311 w416 w584 w607]
      tunnel: w275 -> [w293 w310 w415 w583 _]
      tunnel: [w286 w323 w425 w588 w607] -> w270
      tunnel: [w293 w320 w424 w587 w606] -> w269
      tunnel: w260 -> [w290 w324 w441 _ w609]
      tunnel: "Save Volume" -> [_ w319 _ _ _]
      tunnel: w262 -> [_ _ w405 _ _]
      tunnel: w261 -> [_ _ w383 _ _]
      frame 0, Default {
        n185 = call-dynamic "Read FPGA VI Reference.vi"("AODAcq in"=w286) -> ("FPGA VI Reference"=w277:T8)  [unwired: 8 in, 2 out]
        n186 = Unbundle(w290) -> ("queue out"=w289:refnum<queue>, "queue out"=w288:refnum<queue>, "queue out"=w287:refnum<queue>)
        n187 = shared-variable "My Computer\\AODAcq.lvclass\\ReadFraction"(0.0 ("ReadFraction")) -> ()  [unwired: 1 in, 1 out]
        n188 = Wait (ms)(milliseconds to wait=u32 50) -> ()  [unwired: 1 out]
        n189 = Flush Queue(queue=w289) -> ()  [unwired: 1 in, 3 out]
        n190 = Flush Queue(queue=w288) -> ()  [unwired: 1 in, 3 out]
        n191 = Flush Queue(queue=w287) -> ()  [unwired: 1 in, 3 out]
        n192 = xnode "Invoke Method"("FPGA VI Reference In"=w277, "Number of Elements"=u32 0) -> ("Elements Remaining"=→"Motion samples remaining")  [unwired: 2 in, 3 out]
        n193 = xnode "Invoke Method"("FPGA VI Reference In"=w277, "Number of Elements"=u32 0) -> ("Elements Remaining"=→"Image samples remaining")  [unwired: 2 in, 3 out]
        n194 = xnode "Invoke Method"("FPGA VI Reference In"=w277, "Number of Elements"=u32 0) -> ("Elements Remaining"=→"Raw samples remaining")  [unwired: 2 in, 3 out]
        n195 = xnode "Invoke Method"("FPGA VI Reference In"=w277, "Number of Elements"=u32 0) -> ("Elements Remaining"=→"Temporal samples remaining")  [unwired: 2 in, 3 out]
        "Finished" <- FALSE ("Finished")
      }
      frame 1 {
        w303 = 2 ("dimension size")
        # "Volume imaging mode"
        n196 = local write "Volume"(FALSE ("Volume")) -> ()
        n197 = local write "Tab Control"(enum32{"Setup", "Volume", "Traces"}."Volume" ("Tab Control")) -> ()
        n198 = case shown="\"20x Olympus\", Default" "Objective" {
          tunnel: [T2 {"XStart"=1460000, "XEnd"=1460000, "XNum"=1, "YStart"=1460000, "YEnd"=1460000, "YNum"=1, "ZStart"=700, "ZEnd"=700, "ZNum"=1} ("y")] -> w339
          tunnel: [20] -> w296
          frame "20x Olympus", Default {
          }
        }
        "Lens Magnification" <- w296
        n199 = call "GetObjectivePosition.vi"() -> ("output cluster"=w297:cluster{"X":dbl, "Y":dbl, "Z":dbl})  [unwired: 8 in, 3 out]
        "Objective Position" <- w297
        n200 = call-dynamic "Init.vi"("error in (no error)"=w310, "Channel"=i16 3, "AODAcq in"=w311) -> ("error out"=w309:errorcluster, "AODAcq out"=w308:refnum<class "AODAcq.lvclass">)  [unwired: 7 in]
        n201 = call-dynamic "Reset.vi"("error in (no error)"=w309, "AODAcq in"=w308) -> ("error out"=w300:errorcluster, "AODAcq out"=w301:refnum<class "AODAcq.lvclass">)  [unwired: 8 in]
        n202 = call-dynamic "Write Object Position.vi"("error in (no error)"=w300, "Object Position"=w297, "AODAcq in"=w301) -> ("error out"=w298:errorcluster, "AODAcq out"=w299:refnum<class "AODAcq.lvclass">)  [unwired: 7 in]
        n203 = Multiply(x=w339, y="Scan Settings (um)") -> (x*y=w342:T2)
        "Scan Settings" <- w342
        n204 = Unbundle By Name("Scan Settings (um)") -> ("XNum"=w341:i32, "YNum"=w340:i32, "ZNum"=w305:i32)
        n205 = call-dynamic "Configure Volume.vi"("Save"=w319, "error in (no error)"=w298, "NumReps"="Volume Reps", "Scan Settings"=w342, "AODAcq in"=w299) -> ("error out"=w327:errorcluster, "AODAcq out"=w328:refnum<class "AODAcq.lvclass">)  [unwired: 5 in]
        n206 = call-dynamic "Start.vi"("error in (no error)"=w327, "AODAcq in"=w328) -> ("error out"=w315:errorcluster, "AODAcq out"=w317:refnum<class "AODAcq.lvclass">)  [unwired: 8 in]
        n207 = Select(t=w305, s="Disp Volume", f=u32 1) -> (s? t:f=w304:u32)
        n208 = call-dynamic "Read Recording File.vi"("error in (no error)"=w315, "AcquistionObject in"=w317) -> ("error out"=w314:errorcluster, "Recording File"=→"Recording File":path, "AcquistionObject out"=w316:refnum<class "AODAcq.lvclass">)  [unwired: 7 in]
        n209 = Compound Arithmetic op=MULTIPLY(w341, w340, w304) -> (w302:u32)
        n210 = call-dynamic "Read FPGA VI Reference.vi"("error in (no error)"=w314, "AODAcq in"=w316) -> ("error out"=w325:errorcluster, "FPGA VI Reference"=w331:T8, "AODAcq out"=w326:refnum<class "AODAcq.lvclass">)  [unwired: 7 in]
        n211 = Unbundle(w324) -> ("queue out"=w332:refnum<queue>, "queue out"=w329:refnum<queue>)  [unwired: 1 out]
        n212 = Initialize Array(0, w303, w302) -> (w338:i32[][])
        n213 = call-dynamic "Read Loop.vi"("error in (no error)"=w325, "ReadElements"="VolumeElements", "Queues"=w324, "AODAcq in"=w326) -> ("error out"=w321:errorcluster, "AODAcq out"=w322:refnum<class "AODAcq.lvclass">)  [unwired: 6 in]
        n214 = while {
          tunnel: w332 -> [w363]
          shift-right: [w359] -> _
          shift-left: w338 -> [w348]
          shift-right: [w360] -> _
          shift-left: 0 -> [w361]
          tunnel: w302 -> [w358]
          tunnel: 1000 ("timeout in ms (-1)") -> [w357]
          tunnel: w331 -> [w354]
          tunnel: w329 -> [w352]
          tunnel: w303 -> [w350]
          tunnel: w302 -> [w349]
          stop <- w355 stop-if-true
          n215 = Flush Queue(queue=w352) -> ()  [unwired: 1 in, 3 out]
          n216 = Reshape Array(w348, w349, w350) -> ()  [unwired: 1 out]
          n217 = local read "Abort"() -> (w351:bool)
          n218 = shared-variable "My Computer\\AODAcq.lvclass\\ScanFraction"() -> (w353:dbl)  [unwired: 1 in, 1 out]
          n219 = shared-variable "My Computer\\AODAcq.lvclass\\ReadFraction"() -> (→"Progress":dbl)  [unwired: 1 in, 1 out]
          n220 = xnode "Read/Write Control"("FPGA VI Reference In"=w354, "Control.Abort"=w351) -> ()  [unwired: 1 in, 2 out]
          n221 = Dequeue Element(queue=w363, timeout in ms (-1)=w357) -> (element=w362:waveform(i32)[], timed out?=w347:bool)  [unwired: 1 in, 2 out]
          n222 = case shown="True" w347 {
            tunnel: w348 -> [w369 w378]
            tunnel: w362 -> [w368 _]
            tunnel: w361 -> [w367 w377]
            tunnel: [w366 w377] -> w360
            tunnel: [w365 w378] -> w359
            tunnel: w358 -> [w364 _]
            tunnel: [_ w376] -> w355
            frame False {
              n223 = for {
                tunnel: w369 -> [w373] mode=indexing
                tunnel: w368 -> [w375] mode=indexing
                tunnel: [w374] -> w365 mode=indexing
                tunnel: w367 -> [w371]
                tunnel: [w372] -> w366
                tunnel: w364 -> [_]
                n224 = Unbundle By Name(w375) -> ("Y"=w370:i32[])
                n225 = call "WraparoundUpdate.vi"("Data"=w370, "Location"=w371, "Accumulator"=w373) -> ("NewLocation"=w372:u32, "Accumulated"=w374:i32[])  [unwired: 7 in]
              }
            }
            frame True {
              n226 = local read "Finished"() -> (w376:bool)
            }
          }
          "VolData" <- w359
          n227 = local write "ScanProgress"(w353) -> ()
        }
        n228 = flat-sequence {
          tunnel: w321 -> [_]
          tunnel: [FALSE] -> w318
          frame #0 {
            n229 = local write "Finished"(TRUE ("Finished")) -> ()
          }
        }
        n230 = call-dynamic "Stop.vi"("error in (no error)"=w321, "AODAcq in"=w322) -> ("error out"=w320:errorcluster, "AODAcq out"=w323:refnum<class "AODAcq.lvclass">)  [unwired: 8 in]
        n231 = local write "Save Volume"(w318) -> ()
      }
      frame 2 {
        (unwired) 0
        # "Point imaging mode"
        n232 = global write "GlobalVars.vi" "Scanning"(TRUE ("Scanning")) -> ()
        n233 = local write "Scan"(FALSE ("Scan")) -> ()
        n234 = Flush Queue(queue=w383) -> (queue out=w382:refnum<queue>)  [unwired: 1 in, 2 out]
        n235 = call-dynamic "Init.vi"("error in (no error)"=w415, "Channel"=i16 3, "AODAcq in"=w416) -> ("error out"=w410:errorcluster, "AODAcq out"=w407:refnum<class "AODAcq.lvclass">)  [unwired: 7 in]
        n236 = call "GetObjectivePosition.vi"() -> ("output cluster"=w406:cluster{"X":dbl, "Y":dbl, "Z":dbl})  [unwired: 8 in, 3 out]
        n237 = local read "Scan Settings (um)"() -> (w391:T2)
        n238 = local read "Number selected"() -> (w397:u32)
        n239 = local write "Tab Control"(enum32{"Setup", "Volume", "Traces"}."Traces" ("Tab Control")) -> ()
        n240 = local write "Objective Position"(w406) -> ()
        n241 = call-dynamic "Write Object Position.vi"("error in (no error)"=w410, "Object Position"=w406, "AODAcq in"=w407) -> ("error out"=w409:errorcluster, "AODAcq out"=w408:refnum<class "AODAcq.lvclass">)  [unwired: 7 in]
        n242 = local read "Scan Settings"() -> (w392:T2)
        n243 = call-dynamic "Reset.vi"("error in (no error)"=w409, "AODAcq in"=w408) -> ("error out"=w450:errorcluster, "AODAcq out"=w403:refnum<class "AODAcq.lvclass">)  [unwired: 8 in]
        n244 = local read "Motion Points (Ch1)"() -> (w390:u32)
        n245 = local read "Motion rate (Hz)"() -> (w393:dbl)
        n246 = local read "Motion ROIs"() -> (w396:T1)
        n247 = local read "GridPoints"() -> (w394:u16)
        n248 = call-dynamic "ConfigurePerCellMotionAnalysis.vi"("Scan Settings (um)"=w391, "Points Selected"=w397, "Scan Settings"=w392, "Sampling Structure"="Sampling Structure", "Per Cell Motion Analysis"="Per Cell Motion Analysis", "In Points"="Points", "AODAcq in"=w403) -> ("Additional Points"=w400:i32, "Out Points"=w395:i32[][])  [unwired: 1 in, 2 out]
        n249 = case shown="True" "Per Cell Motion Analysis" {
          tunnel: w397 -> [w451 w455]
          tunnel: w400 -> [_ w454]
          tunnel: [w451 w452] -> w399
          frame False {
          }
          frame True {
            n250 = Multiply(x=w455, y=w454) -> (x*y=w453:u32)
            n251 = Add(x=w455, y=w453) -> (x+y=w452:u32)
          }
        }
        n252 = call "AutoConfigureAdditionalMotionPlanes.vi"("Motion ROIs"=w396, "Number of Motion Points"=w390, "Plane Params"="Motion Box Params", "In Points"=w395, "Grid Points"=w394, "Motion Rate (Hz)"=w393, "Scan Settings"=w392, "Scan Settings (um)"=w391) -> ("X-Y Motion Points"=w386:i32[][], "Out Points"=w388:i32[][], "Total Motion Points"=w389:i32, "Motion Increment"=w387:i32, "Y-Z Motion Points"=w385:i32[][])  [unwired: 1 in, 2 out]
        "Out Points" <- w388
        "Total Motion Points" <- w389
        n253 = local read "GridPoints"() -> (w434:u16)
        n254 = Initialize Array(0 ("element"), w389) -> ()  [unwired: 1 out]
        n255 = Quotient & Remainder(x=w389, y=w434) -> (floor(x/y)=w435:i32)  [unwired: 1 out]
        n256 = local write "X-Y Motion Points"(w386) -> ()
        n257 = local write "Motion Increment"(w387) -> ()
        n258 = local write "Y-Z Motion Points"(w385) -> ()
        n259 = Multiply(x="Scan Time (s)", y=50000.0) -> (x*y=w447:dbl)
        n260 = Decrement(x=w387) -> (x-1=w428:i32)
        n261 = Divide(x=w447, y=w399) -> (x/y=w430:dbl)
        n262 = Divide(x=w428, y=w387) -> (x/y=w427:dbl)
        n263 = Quotient & Remainder(x="TraceElements", y=w399) -> (floor(x/y)=w443:u32)  [unwired: 1 out]
        n264 = Multiply(x=w399, y=w443) -> (x*y=w442:u32)
        n265 = Multiply(x=w427, y=w430) -> (x*y=w429:dbl)
        n266 = call-dynamic "Configure PointScan.vi"("AODAcq in"=w403, "Save"=TRUE ("Save Volume"), "Store Raw"="Store Raw", "Points"=w388, "GridSize"=w394, "Reps"=w429, "error in (no error)"=w450, "Motion Points"=w389, "Motion Increment"=w387) -> ("AODAcq out"=w438:refnum<class "AODAcq.lvclass">, "error out"=w439:errorcluster)  [unwired: 5 in]
        n267 = Unbundle(w441) -> ("queue out"=w440:refnum<queue>, "queue out"=w436:refnum<queue>)  [unwired: 1 out]
        n268 = call-dynamic "Read FPGA VI Reference.vi"("error in (no error)"=w439, "AODAcq in"=w438) -> ("error out"=w423:errorcluster, "FPGA VI Reference"=w437:T8, "AODAcq out"=w422:refnum<class "AODAcq.lvclass">)  [unwired: 7 in]
        n269 = call-dynamic "Start.vi"("error in (no error)"=w423, "AODAcq in"=w422) -> ("error out"=w419:errorcluster, "AODAcq out"=w421:refnum<class "AODAcq.lvclass">)  [unwired: 8 in]
        n270 = while {
          tunnel: w399 -> [w496]
          tunnel: 300 ("timeout in ms (-1)") -> [w486]
          tunnel: w443 -> [w491]
          tunnel: w440 -> [w489]
          tunnel: w437 -> [w488]
          tunnel: w436 -> [w482]
          tunnel: w435 -> [_]
          tunnel: w434 -> [w469]
          border: 0 -> [_]
          tunnel: w405 -> [w478]
          tunnel: w389 -> [w461]
          tunnel: w382 -> [w464]
          shift-right: [w458] -> _
          shift-left: 0 -> [w459]
          i -> [w481]
          stop <- w475 stop-if-true
          n271 = Increment "Loop Counter"(x=w459) -> (x+1=w458:i32)
          n272 = Dequeue Element(queue=w489, timeout in ms (-1)=w486) -> (element=w500:waveform(i32)[])  [unwired: 1 in, 3 out]
          n273 = Dequeue Element(queue=w482, timeout in ms (-1)=w486) -> (element=w477:waveform(i32)[])  [unwired: 1 in, 3 out]
          n274 = local read "Finished"() -> (w479:bool)
          n275 = shared-variable "My Computer\\AODAcq.lvclass\\ReadFraction"() -> (w484:dbl)  [unwired: 1 in, 1 out]
          n276 = shared-variable "My Computer\\AODAcq.lvclass\\ScanFraction"() -> (→"ScanProgress":dbl)  [unwired: 1 in, 1 out]
          n277 = Divide(x=50000, y=w496) -> (x/y=w495:dbl)
          n278 = xnode "Read/Write Control"("FPGA VI Reference In"=w488, "Control.Abort"="Abort") -> ()  [unwired: 1 in, 2 out]
          n279 = Divide(x=w495, y="Down Rate") -> (x/y=w498:dbl)
          n280 = Not Equal To 0?(x=w481) -> (x != 0?=w480:bool)
          n281 = Round To Nearest(number=w498) -> (nearest integer value=w493:dbl)
          n282 = Square(x=w469) -> (x^2=w460:u16)
          n283 = And(x=w479, y=w480) -> (x .and. y?=w475:bool)
          n284 = local write "Progress"(w484) -> ()
          n285 = Divide(x=w461, y=w460) -> (x/y=w472:dbl)
          n286 = Decrement(x="Motion Channel To Analyze") -> (x-1=w473:i32)
          n287 = Multiply(x=w460, y=u16 2) -> (x*y=w467:u16)
          n288 = In Range and Coerce(upper limit=w491, x=w493, lower limit=1.0) -> (coerced(x)=w490:dbl)  [unwired: 1 out]
          n289 = case shown="\"Traces\"" "Tab Control" {
            tunnel: w496 -> [_ w561]
            tunnel: w500 -> [_ w567]
            tunnel: w490 -> [_ w564]
            frame Default {
            }
            frame "Traces" {
              n290 = Index Array(array=w567, index=0) -> (element=w548:waveform(i32))
              n291 = Add(x=w548, y="Baseline Offset") -> (x+y=w546:waveform(dbl))
              n292 = Unbundle By Name(w546) -> ("dt"=w569:dbl, "Y"=w566:dbl[])
              n293 = Multiply(x=w561, y=w569) -> (x*y=w568:dbl)
              n294 = Array Size(array=w566) -> (size(s)=w556:i32)
              n295 = Divide(x=w556, y=w561) -> (x/y=w560:dbl)
              n296 = feedback #1() -> (w555:i32)
              n297 = Add(x=w556, y=w555) -> (x+y=w551:i32)
              n298 = feedback-in #1(w551) -> ()
              n299 = Reshape Array(w566, w560, w561) -> (w559:dbl[][])
              n300 = Less?(x=w551, y=50000) -> (x < y?=w549:bool)
              n301 = Transpose 2D Array(2D array=w559) -> (transposed array=w558:dbl[][])
              n302 = for {
                tunnel: w568 -> [w580]
                tunnel: w546 -> [w579]
                tunnel: [w578] -> w563 mode=indexing
                tunnel: w558 -> [w577] mode=indexing
                n303 = Bundle By Name(cluster=w579, "dt"=w580, "Y"=w577) -> (w578:waveform(dbl))
              }
              n304 = Select(t=1.0, s=w549, f=0.001 ("Baseline Rate")) -> (s? t:f=w552:dbl)
              n305 = case shown="True" "Decimate" {
                tunnel: "Spacing" -> [_ w576]
                tunnel: w564 -> [_ w575]
                tunnel: w563 -> [w571 w574]
                tunnel: [w571 w573] -> w562
                tunnel: w552 -> [_ w572]
                frame False {
                }
                frame True {
                  n306 = call "CleanupTraces.vi"("Baseline Rate"=w572, "Spacing"=w576, "decimating factor"=w575, "Traces in"=w574) -> ("Traces out"=w573:waveform(dbl)[])  [unwired: 7 in]
                }
              }
              "Traces" <- w562
            }
          }
          n307 = Index Array(array=w477, index=w473) -> (element=w485:waveform(i32))
          n308 = Not(x=w475) -> (.not. x?=w476:bool)
          n309 = Divide(x=w472, y=2.0) -> (x/y=w470:dbl)
          n310 = Increment(x=w470) -> (x+1=w466:dbl)
          n311 = Unbundle By Name(w485) -> ("Y"=w457:i32[])
          n312 = global write "GlobalVars.vi" "Scanning"(w476) -> ()
          n313 = call "Motion FIFO.vi"("Packet Length"=w461, "Data"=w457, "Motion FIFO"=w464) -> ("Number of Packets"=w463:i32, "Array"=w462:i32[])  [unwired: 7 in]
          n314 = Multiply(x=w466, y=w460) -> (x*y=w465:dbl)
          n315 = for {
            N: w463 -> [_]
            tunnel: w478 -> [w515]
            tunnel: w469 -> [w513]
            tunnel: w467 -> [w512]
            tunnel: w465 -> [w511]
            tunnel: w462 -> [w510]
            tunnel: w461 -> [w502]
            tunnel: w460 -> [w501]
            i -> [w509]
            n316 = Multiply(x=w502, y=w509) -> (x*y=w508:i32)
            n317 = Array Subset(array=w510, index=w508, length=w502) -> (w507:i32[])
            n318 = Array Subset(array=w507, index=w501, length=w501) -> (w503:i32[])
            n319 = Array Subset(array=w507, index=w511, length=w501) -> (w504:i32[])
            n320 = Reshape Array(w503, w513, w513) -> (w506:i32[][])
            n321 = Reshape Array(w504, w513, w513) -> (w514:i32[][])
            n322 = Insert Into Array(array=w506, new element=w514) -> (w505:i32[][])  [unwired: 2 in]
            n323 = local read "Motion Ch1"() -> (w518:T4)
            n324 = case shown="True" "Motion Analysis" {
              tunnel: w513 -> [_ w538]
              tunnel: w515 -> [_ w537]
              tunnel: w505 -> [_ w536]
              tunnel: w501 -> [_ w535]
              tunnel: w512 -> [_ w534]
              frame False {
                n325 = global read "GlobalVars.vi" "VI Open"() -> (w520:bool)
                n326 = case shown="True" w520 {
                  frame False {
                  }
                  frame True {
                    n327 = global write "GlobalVars.vi" "VI Open"(FALSE ("VI Open")) -> ()
                    n328 = vi-ref "RunDuringExperiment.vi"() -> (w522:refnum<vi>)
                    n329 = invoke on="Invoke Node" class="VI" method="Abort VI"(reference=w522) -> (reference out=w523:refnum<vi>)  [unwired: 2 in, 2 out]
                    n330 = invoke class="VI" method="FP.Close"(reference=w523) -> ()  [unwired: 2 in, 3 out]
                  }
                }
              }
              frame True {
                n331 = local read "Scan Settings (um)"() -> (w530:T2)
                n332 = local read "Y-Z Motion Points"() -> (w527:i32[][])
                n333 = local read "X-Y Motion Points"() -> (w528:i32[][])
                n334 = local read "Scan Settings"() -> (w531:T2)
                n335 = Bundle("Scan Settings"=w531, "Scan Settings (um)"=w530) -> (w529:T9)  [unwired: 1 in]
                n336 = Array Subset(array=w527, index (row)=w535, length (row)=w535) -> (w525:i32[][])  [unwired: 2 in]
                n337 = Array Subset(array=w528, index (row)=w535, length (row)=w535) -> (w526:i32[][])  [unwired: 2 in]
                n338 = global read "GlobalVars.vi" "VI Open"() -> (w524:bool)
                n339 = call "InterfaceAODSWWithStabilizationSW.vi"("Y-Z Motion Points"=w525, "X-Y Motion Points"=w526, "Grid Points"=w538, "Motion Points"=w534, "Scan Info"=w529, "Data"=w536) -> ("Number of Planes"=w533:dbl, "Array"=w532:cluster{dbl[][], dbl, dbl, dbl, dbl, dbl, dbl}[])  [unwired: 4 in]
                n340 = stacked-sequence {
                  tunnel: w533 -> [w543 _]
                  tunnel: w537 -> [_ w545]
                  tunnel: w532 -> [_ w544]
                  frame #0 {
                    n341 = global write "GlobalVars.vi" "Number of Scan Planes"(w543) -> ()
                  }
                  frame #1 {
                    n342 = Lossy Enqueue Element(queue=w545, element=w544) -> ()  [unwired: 1 in, 4 out]
                  }
                }
                n343 = case shown="False" w524 {
                  frame False {
                    n344 = vi-ref "RunDuringExperiment.vi"() -> (w542:refnum<vi>)
                    n345 = invoke on="Invoke Node" class="VI" method="FP.Open"(reference=w542) -> (reference out=w541:refnum<vi>)  [unwired: 4 in, 4 out]
                    n346 = invoke class="VI" method="Run VI"(reference=w541, "Wait until done"=FALSE ("Wait Until Done"), "Auto Dispose Ref"=TRUE ("Auto Dispose Reference")) -> ()  [unwired: 2 in, 5 out]
                  }
                  frame True {
                  }
                }
              }
            }
            n347 = To Single Precision Float(number=w505) -> (single precision float=w517:sgl[][])
            n348 = call "IMAQ ArrayToImage"("Image Pixels (Float)"=w517, "Image"=w518) -> ("Image Out"=w519:T4)  [unwired: 8 in, 1 out]
            n349 = local write "Motion Ch1"(w519) -> ()
          }
        }
        n350 = call-dynamic "Read Recording File.vi"("error in (no error)"=w419, "AcquistionObject in"=w421) -> ("error out"=w413:errorcluster, "Recording File"=w418:path, "AcquistionObject out"=w420:refnum<class "AODAcq.lvclass">)  [unwired: 7 in]
        n351 = local write "Recording File"(w418) -> ()
        n352 = call-dynamic "Read Loop.vi"("error in (no error)"=w413, "ReadElements"=w442, "Queues"=w441, "AODAcq in"=w420) -> ("error out"=w412:errorcluster, "AODAcq out"=w426:refnum<class "AODAcq.lvclass">)  [unwired: 6 in]
        n353 = flat-sequence {
          tunnel: w412 -> [_]
          frame #0 {
            n354 = local write "Finished"(TRUE ("Finished")) -> ()
          }
        }
        n355 = call-dynamic "Stop.vi"("error in (no error)"=w412, "AODAcq in"=w426) -> ("error out"=w424:errorcluster, "AODAcq out"=w425:refnum<class "AODAcq.lvclass">)  [unwired: 8 in]
      }
      frame 4 {
        n356 = call-dynamic "Reset.vi"("error in (no error)"=w583, "AODAcq in"=w584) -> ("error out"=w582:errorcluster, "AODAcq out"=w581:refnum<class "AODAcq.lvclass">)  [unwired: 8 in]
        n357 = call-dynamic "Read FPGA VI Reference.vi"("error in (no error)"=w582, "AODAcq in"=w581) -> ("error out"=w590:errorcluster, "FPGA VI Reference"=w591:T8, "AODAcq out"=w589:refnum<class "AODAcq.lvclass">)  [unwired: 7 in]
        n358 = flat-sequence {
          tunnel: w591 -> [w594]
          tunnel: w590 -> [w592]
          tunnel: w589 -> [w593]
          tunnel: [w593] -> w586
          tunnel: [w592] -> w585
          tunnel: [w596] -> w587
          tunnel: [w595] -> w588
          tunnel: w586 -> [w598]
          tunnel: w585 -> [w597]
          frame #0 {
            n359 = call "SweepSettings.vi"("FPGA VI Reference Out"=w594) -> ()  [unwired: 11 in]
          }
          frame #1 {
            n360 = call-dynamic "GetStatus.vi"("error in (no error)"=w597, "AODAcq in"=w598) -> ("error out"=w596:errorcluster, "AODAcq out"=w595:refnum<class "AODAcq.lvclass">)  [unwired: 7 in, 1 out]
          }
        }
      }
      frame 8 {
        n361 = Unbundle(w609) -> ("queue out"=w603:refnum<queue>)  [unwired: 2 out]
        n362 = local write "Ephys"(FALSE ("Ephys")) -> ()
        n363 = local write "Ephys"(TRUE ("Ephys")) -> ()
        n364 = local write "Tab Control"(enum32{"Setup", "Volume", "Traces", "Motion"}."Traces" ("Tab Control")) -> ()
        n365 = call "DAQ Assistant"() -> ("task out"=w610:refnum<k21>, "error out"=w605:errorcluster)  [unwired: 16 in, 2 out]
        n366 = while {
          tunnel: w610 -> [w619]
          tunnel: w603 -> [w618]
          tunnel: [w617] -> w608
          tunnel: w605 -> [w616]
          tunnel: [w614] -> w604
          tunnel: [FALSE ("Ephys")] -> w600
          stop <- w620 stop-if-true
          n367 = call-poly <vilib>:"DAQmx Read.vi"("task/channels in"=w619, "error in"=w616) -> ("task out"=w617:refnum<k21>, "data"=w612:waveform(dbl), "error out"=w615:errorcluster)  [unwired: 11 in]
          "Waveform Chart" <- w612
          n368 = Build Array(w612) -> (w611:waveform(dbl)[])
          n369 = Enqueue Element(queue=w618, element=w611, error in (no error)=w615) -> (error out=w614:errorcluster)  [unwired: 1 in, 2 out]
          n370 = local read "Abort"() -> (w620:bool)
        }
        "Ephys" <- w600
        n371 = call <vilib>:"DAQmx Clear Task.vi"("task in"=w608, "error in"=w604) -> ("error out"=w606:errorcluster)  [unwired: 13 in]
      }
    }
    "AODAcq out" <- w270
    n372 = call <vilib>:"Simple Error Handler.vi"("error in (no error)"=w269) -> ("error out"=w268:errorcluster)  [unwired: 4 in, 4 out]
    "Volume" <- "Volume"
    "Scan" <- "Scan"
    "Numeric" <- w263
  }
  "Stopped" <- w10
  n373 = case shown="True" w10 {
    tunnel: [errorcluster {"status"=FALSE, "code"=0, "source"=""} ("error out") w623] -> w11
    frame False {
    }
    frame True {
      n374 = global read "GlobalVars.vi" "VI Open"() -> (w622:bool)
      n375 = case shown="True" w622 {
        tunnel: [errorcluster {"status"=FALSE, "code"=0, "source"=""} ("error out") w627] -> w623
        frame False {
        }
        frame True {
          n376 = vi-ref "RunDuringExperiment.vi"() -> (w625:refnum<vi>)
          n377 = invoke on="Invoke Node" class="VI" method="Abort VI"(reference=w625) -> (reference out=w626:refnum<vi>)  [unwired: 2 in, 2 out]
          n378 = invoke class="VI" method="FP.Close"(reference=w626) -> (error out=w627:errorcluster)  [unwired: 2 in, 2 out]
        }
      }
    }
  }
  n379 = stacked-sequence {
    tunnel: w11 -> [_ w631]
    frame #0 {
      n380 = Wait Until Next ms Multiple(millisecond multiple=u32 100) -> ()  [unwired: 1 out]
    }
    frame #1 {
      n381 = global read "GlobalVars.vi" "MotionAnalysis"() -> (w629:refnum<queue>)
      n382 = local read "Motion FIFO"() -> (w630:refnum<queue>)
      n383 = Release Queue(queue=w629, error in (no error)=w631) -> ()  [unwired: 1 in, 3 out]
      n384 = Release Queue(queue=w630) -> ()  [unwired: 2 in, 3 out]
    }
  }
  "Points_um" <- dbl[][] [] ("Points_um")
